vi "RDS Serial Handle Frame.vi"(8 "error in (no error)":errorcluster, 10 "RDS Serial Frame":refnum<class "RDS Serial Frame.lvclass">, 11 "Depth Instrument in":refnum<class "Depth Instrument.lvclass">) -> (0 "error out":errorcluster, 3 "Depth Instrument out":refnum<class "Depth Instrument.lvclass">)   [LabVIEW 2015, in "Depth Instrument.lvlib" / "Depth Instrument.lvclass"]
uses:
  Depth Instrument.lvclass
  Libraries/RDS Serial Handler/RDS Serial Frame.lvclass
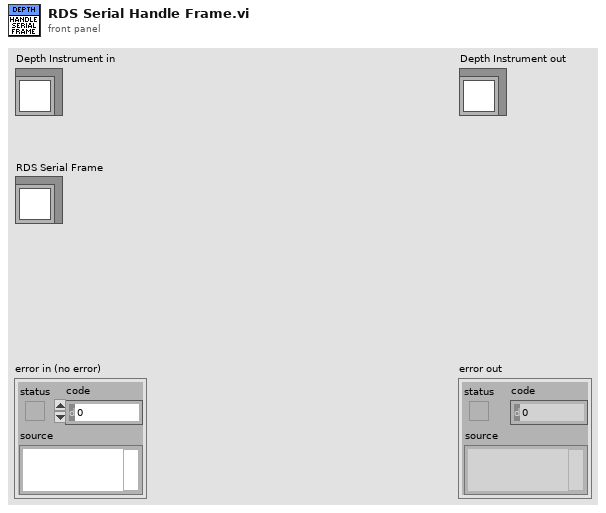
[diagram p1: front panel]
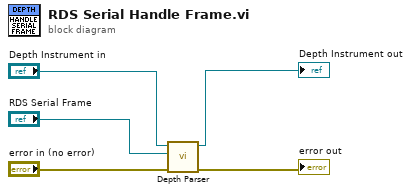
[diagram p0: block diagram]
diagram:
  n1 = call "Depth Parser.vi"("error in (no error)"="error in (no error)", "RDS Serial Frame"="RDS Serial Frame", "Depth Instrument in"="Depth Instrument in") -> ("error out"=→"error out":errorcluster, "Depth Instrument out"=→"Depth Instrument out":refnum<class "Depth Instrument.lvclass">)  [unwired: 7 in]
